vi "Main.vi"() -> ()   [LabVIEW 2015]
doc: "Use this template to build a simple state machine design pattern. Each state executes code and determines which state to transition to."
uses:
  controls/State.ctl
  controls/Data.ctl
  controls/Configuration Settings.ctl
panel:
  out "Current State":string
  out "Data":dbl[](graph)
  in  "Reset Settings":bool
  in  "Clear Graph":bool
  in  "Analyze Data":bool
  in  "Acquire Data":bool
  in  "Configure Data":bool
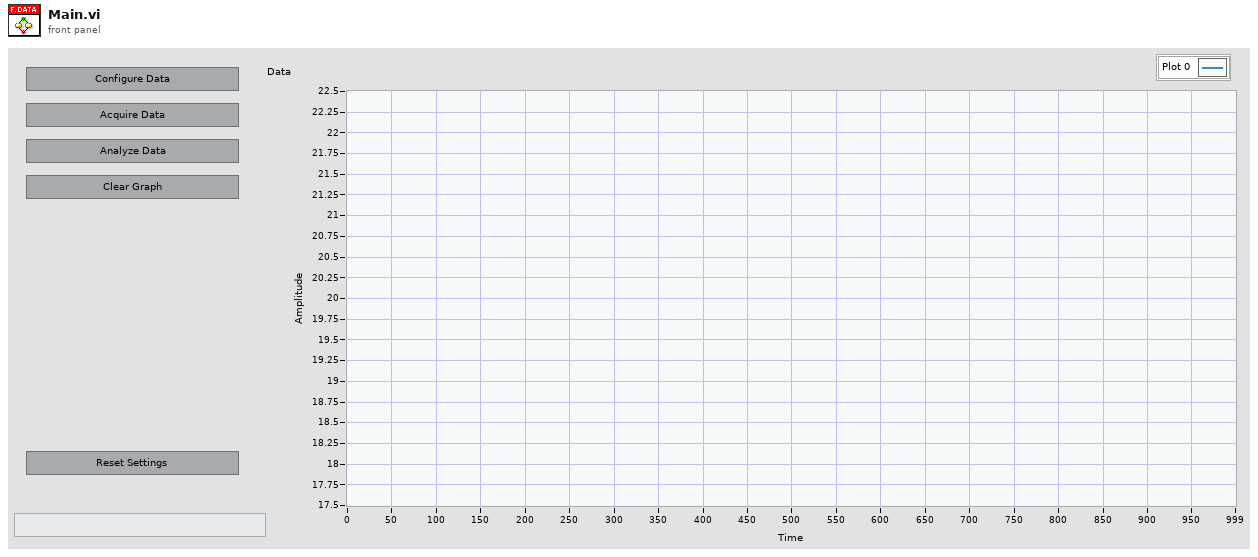
[diagram p1: front panel]
types:
  T1 = typedef "Data.ctl" = cluster{"Configuration Settings":T2, "Data":dbl[]}
  T2 = typedef "Configuration Settings.ctl" = cluster{"Offset":dbl, "Signal Type":enum16{"Sine Wave", "Triangle Wave", "Square Wave", "Sawtooth Wave"}, "Frequency":dbl, "Amplitude":dbl, "Phase":dbl, "Noise Amplitude":dbl}
  T3 = typedef "State.ctl" = enum16{"Initialize", "Wait for Event", "Configure", "Acquire Data", "Update User Interface", "Reset Data", "Clear Data", "Analyse Data", "Stop", "Error"}
  T4 = enum16{"Sine Wave", "Triangle Wave", "Square Wave", "Sawtooth Wave"}
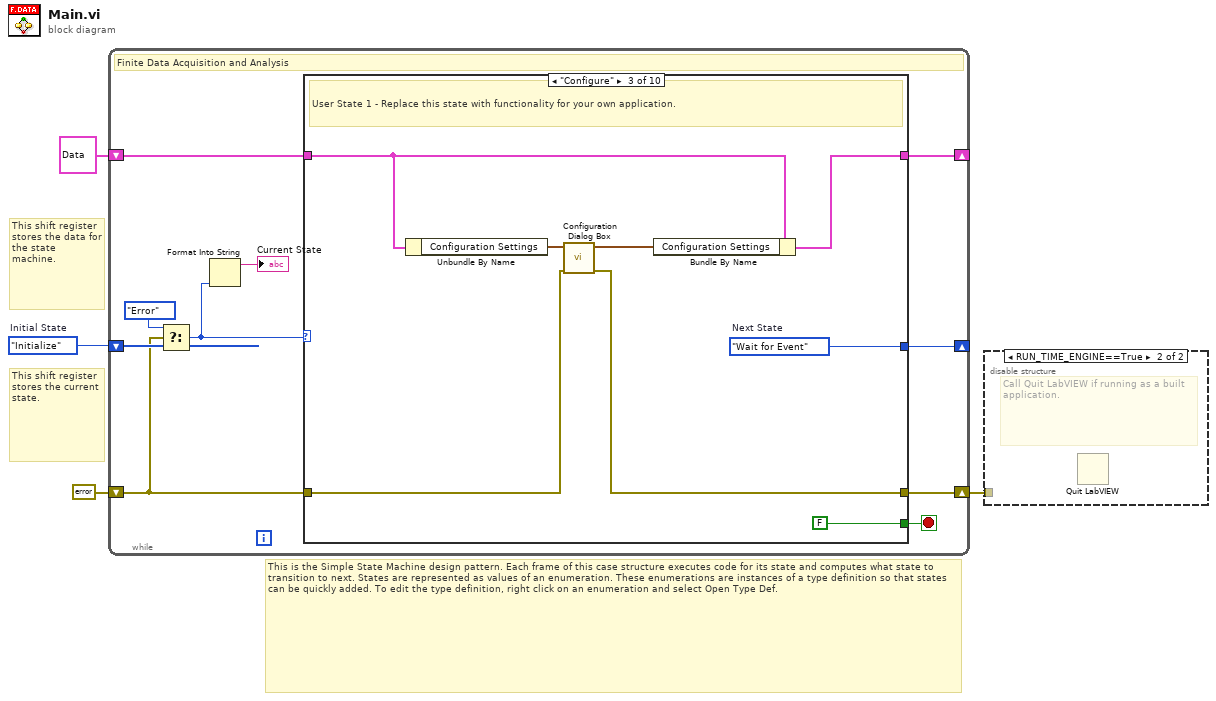
[diagram p0: block diagram]
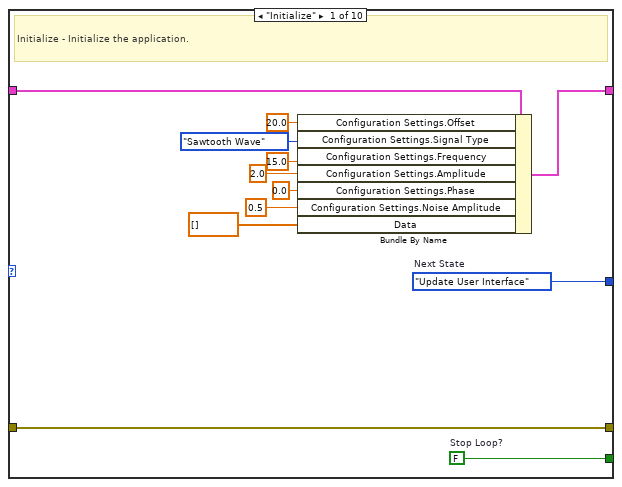
[diagram p3: hidden frame]
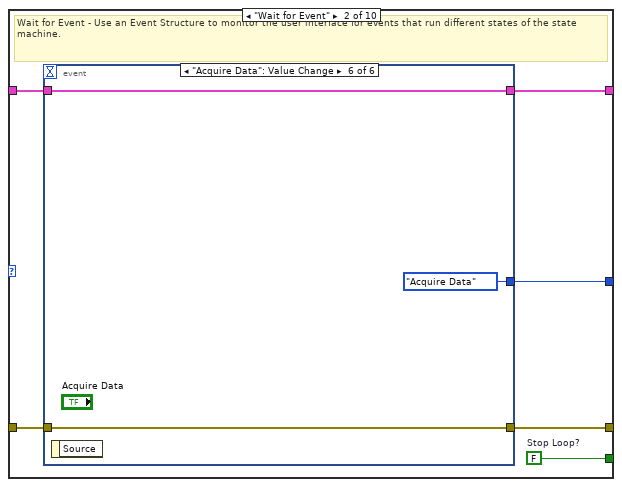
[diagram p4: hidden frame]
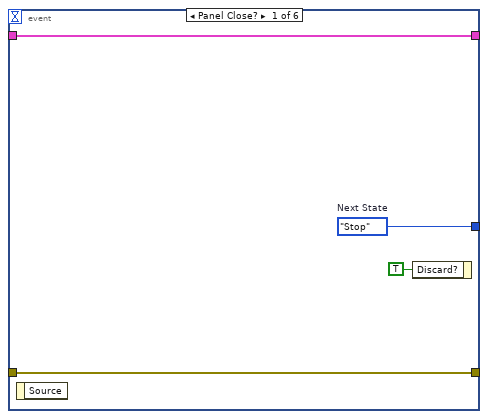
[diagram p5: hidden frame]
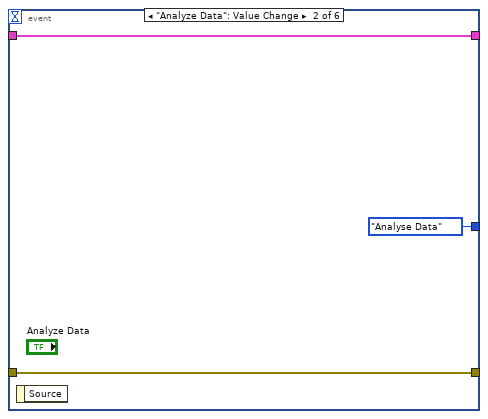
[diagram p6: hidden frame]
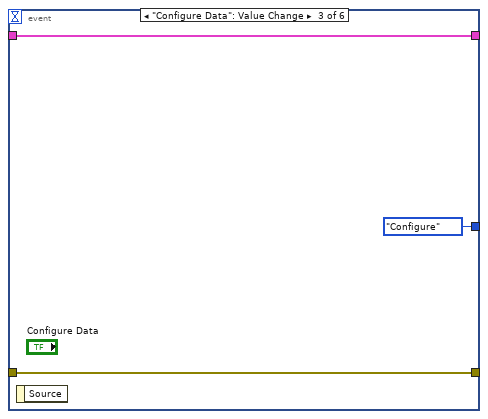
[diagram p7: hidden frame]
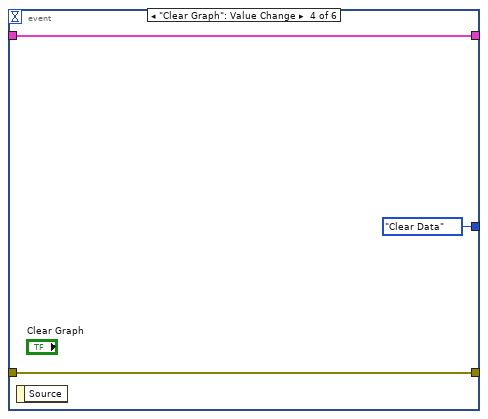
[diagram p8: hidden frame]
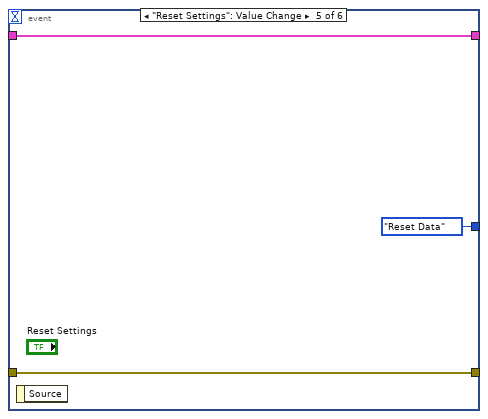
[diagram p9: hidden frame]
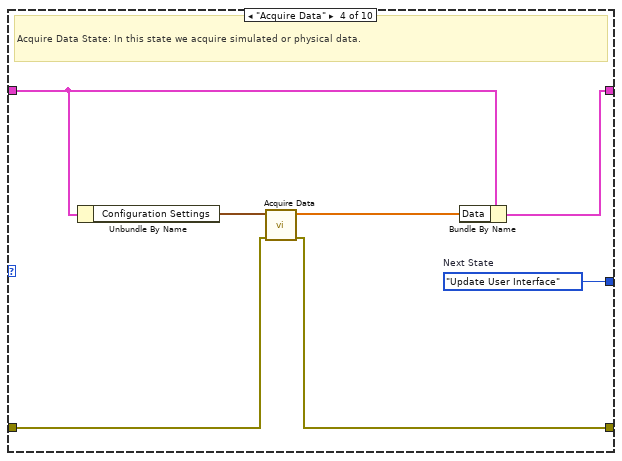
[diagram p10: hidden frame]
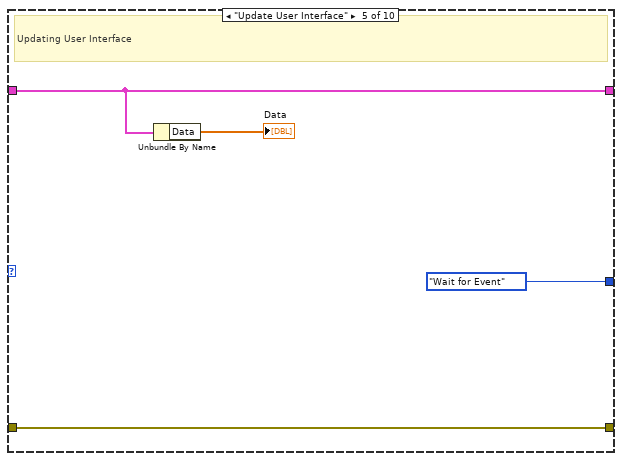
[diagram p11: hidden frame]
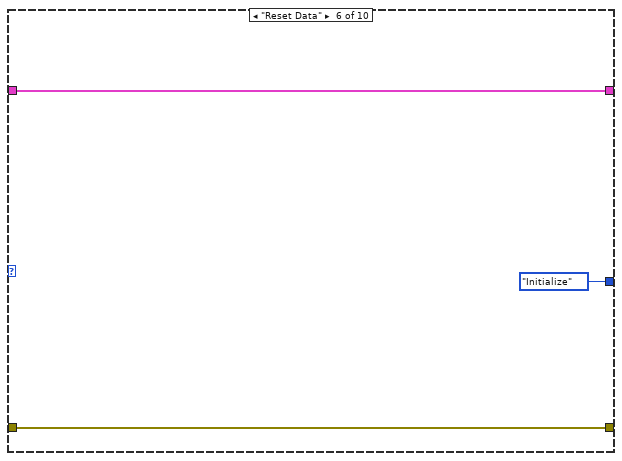
[diagram p12: hidden frame]
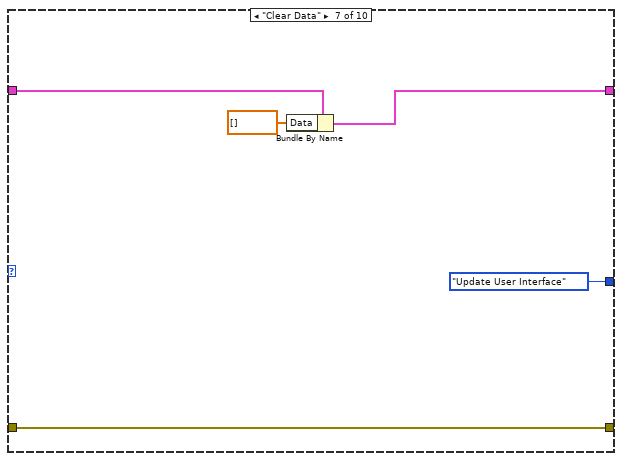
[diagram p13: hidden frame]
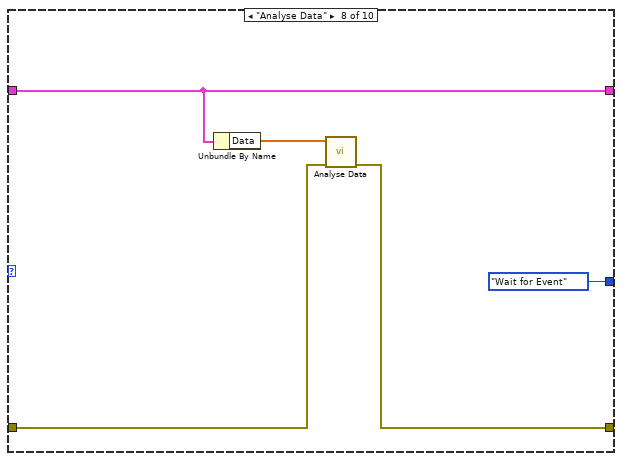
[diagram p14: hidden frame]
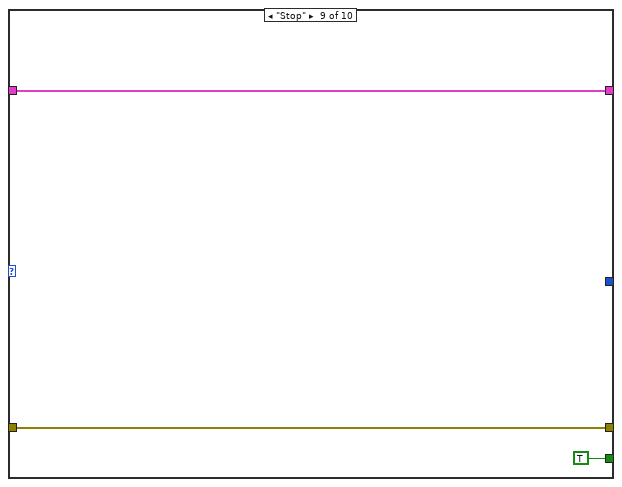
[diagram p15: hidden frame]
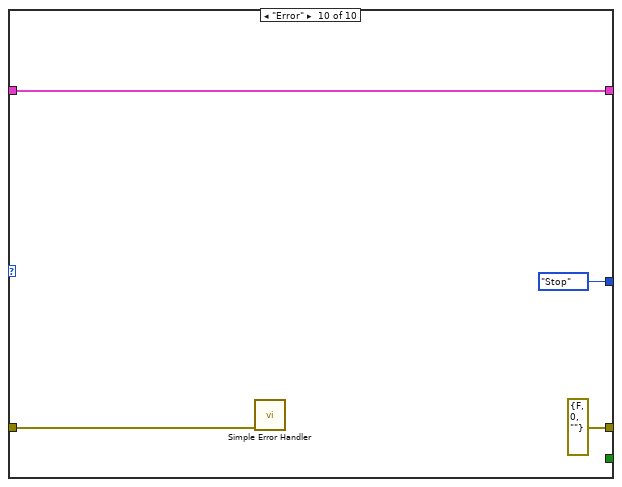
[diagram p16: hidden frame]
diagram:
  w4 = State."Initialize"  # Initial State
  # "This shift register stores the data for the state machine."
  # "This is the Simple State Machine design pattern. Each frame of this case structure executes code for its state and computes what state to transition to next. States are represented as values of an enumeration. These enumerations are instances of a type definition so that states can be quickly added. To edit the type definition, right click on an enumeration and select Open Type Def."
  # "This shift register stores the current state."
  n1 = while {
    shift-right: [w14] -> _
    shift-left: w4 -> [w9]
    shift-right: [w12] -> _
    shift-left: T1 {"Configuration Settings"={"Offset"=0.0, "Signal Type"=enum."Sine Wave", "Frequency"=10.0, "Amplitude"=1.0, "Phase"=0.0, "Noise Amplitude"=1.0}, "Data"=[]} ("Data") -> [w13]
    shift-right: [w11] -> w1
    shift-left: errorcluster {"status"=FALSE, "code"=0, "source"=""} ("error constant") -> [w10]
    stop <- w5 stop-if-true
    # "Finite Data Acquisition and Analysis"
    n2 = Select(t=State."Error", s=w10, f=w9) -> (s? t:f=w7:T3)
    n3 = Format Into String(w7) -> (resulting string=→"Current State":string)  [unwired: 3 in, 1 out]
    n4 = case shown="\"Configure\"" w7 {
      tunnel: [w26 w32 w59 w66 State."Wait for Event" ("(Value Not Used)") State."Initialize" ("(Value Not Used)") State."Update User Interface" ("(Value Not Used)") State."Wait for Event" ("(Value Not Used)") _ State."Stop" ("(Value Not Used)")] -> w14
      tunnel: [w25 w31 FALSE ("Stop Loop?") _ _ _ _ _ TRUE ("Stop Loop?") _] -> w5
      tunnel: w13 -> [w24 w30 w54 w62 w68 w73 w78 w80 w86 w90]
      tunnel: [w23 w29 w52 w60 w68 w73 w75 w80 w86 w90] -> w12
      tunnel: w10 -> [w22 w28 w57 w65 w69 w72 w77 w82 w85 w88]
      tunnel: [w22 w27 w56 w64 w69 w72 w77 w81 w85 errorcluster {"status"=FALSE, "code"=0, "source"=""} ("error constant")] -> w11
      frame "Initialize" {
        w25 = FALSE  # Stop Loop?
        w26 = State."Update User Interface"  # Next State
        # "Initialize - Initialize the application."
        n5 = Bundle By Name(cluster=w24, "Configuration Settings.Offset"=20.0, "Configuration Settings.Signal Type"=T4."Sawtooth Wave", "Configuration Settings.Frequency"=15.0, "Configuration Settings.Amplitude"=2.0, "Configuration Settings.Phase"=0.0, "Configuration Settings.Noise Amplitude"=0.5, "Data"=dbl[] []) -> (w23:T1)
      }
      frame "Wait for Event" {
        w31 = FALSE  # Stop Loop?
        # "Wait for Event - Use an Event Structure to monitor the user interface for events that run different states of the state machine."
        n6 = event shown="[5] \"Acquire Data\": Value Change" {
          selector: _ -> [_ _ _ _ _ _]
          dyn-events: _ -> [_ _ _ _ _ _]
          timeout: _ -> [_ _ _ _ _ _]
          tunnel: [w36 State."Analyse Data" ("Next State") State."Configure" ("Next State") State."Clear Data" ("Next State") State."Reset Data" ("Next State") State."Acquire Data" ("Next State")] -> w32
          tunnel: w30 -> [w35 w39 w42 w45 w48 w51]
          tunnel: [w35 w39 w42 w45 w48 w51] -> w29
          tunnel: w28 -> [w34 w38 w41 w44 w47 w50]
          tunnel: [w34 w38 w41 w44 w47 w50] -> w27
          event Panel Close? {
            w36 = State."Stop"  # Next State
            n7 = event-data() -> ()  [unwired: 1 in, 1 out]
            n8 = event-data("Discard?"=TRUE) -> ()  [unwired: 1 in, 1 out]
          }
          event "Analyze Data": Value Change {
            n9 = event-data() -> ()  [unwired: 1 in, 1 out]
          }
          event "Configure Data": Value Change {
            n10 = event-data() -> ()  [unwired: 1 in, 1 out]
          }
          event "Clear Graph": Value Change {
            n11 = event-data() -> ()  [unwired: 1 in, 1 out]
          }
          event "Reset Settings": Value Change {
            n12 = event-data() -> ()  [unwired: 1 in, 1 out]
          }
          event "Acquire Data": Value Change {
            n13 = event-data() -> ()  [unwired: 1 in, 1 out]
          }
        }
      }
      frame "Configure" {
        w59 = State."Wait for Event"  # Next State
        # "User State 1 - Replace this state with functionality for your own application."
        n14 = Unbundle By Name(w54) -> ("Configuration Settings"=w55:T2)
        n15 = call "Configuration Dialog Box.vi"("error in (no error)"=w57, "Configuration Settings In"=w55) -> ("error out"=w56:errorcluster, "Configuration Settings Out"=w53:T2)  [unwired: 8 in]
        n16 = Bundle By Name(cluster=w54, "Configuration Settings"=w53) -> (w52:T1)
      }
      frame "Acquire Data" {
        w66 = State."Update User Interface"  # Next State
        # "Acquire Data State: In this state we acquire simulated or physical data."
        n17 = Unbundle By Name(w62) -> ("Configuration Settings"=w63:T2)
        n18 = call "Acquire Data.vi"("error in (no error)"=w65, "Configuration Settings"=w63) -> ("error out"=w64:errorcluster, "Data Out"=w61:dbl[])  [unwired: 8 in]
        n19 = Bundle By Name(cluster=w62, "Data"=w61) -> (w60:T1)
      }
      frame "Update User Interface" {
        # "Updating User Interface"
        n20 = Unbundle By Name(w68) -> ("Data"=→"Data":dbl[])
      }
      frame "Reset Data" {
      }
      frame "Clear Data" {
        n21 = Bundle By Name(cluster=w78, "Data"=dbl[] []) -> (w75:T1)
      }
      frame "Analyse Data" {
        n22 = Unbundle By Name(w80) -> ("Data"=w79:dbl[])
        n23 = call "Analyse Data.vi"("error in (no error)"=w82, "Data In"=w79) -> ("error out"=w81:errorcluster)  [unwired: 9 in]
      }
      frame "Stop" {
      }
      frame "Error" {
        n24 = call <vilib>:"Simple Error Handler.vi"("error in (no error)"=w88) -> ()  [unwired: 4 in, 5 out]
      }
    }
  }
  n25 = disable-structure shown="RUN_TIME_ENGINE==True" {
    disable-tunnel: w1 -> [_ _]
    frame condition #0 (active) {
    }
    frame condition #1 {
      # "Call Quit LabVIEW if running as a built application."
      n26 = Quit LabVIEW() -> ()  [unwired: 1 in]
    }
  }
